vi "get_config.vi"(8 "error in":errorcluster) -> (0 "error out":errorcluster, 1 "key":string, 2 "model name":string, 3 "Provider Selector":enum32{"OpenAI", "Gemini"}(ring), 5 "proper config?":bool)   [LabVIEW 2020, in "lv_documentation.lvlib"]
uses:
  lv_documentation.lvlib
  <vilib>/Utility/config.llb/Read Key (String).vi
  <vilib>/Utility/config.llb/NI_LVConfig.lvlib
  <vilib>/httpClient/LabVIEWHTTPClient.lvlib
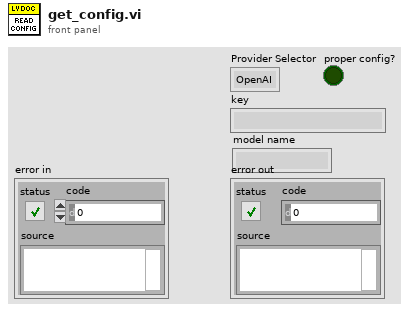
[diagram p1: front panel]
types:
  T1 = typedef "NI_LVConfig.lvlib/Config Data RefNum.ctl" = refnum<k1>
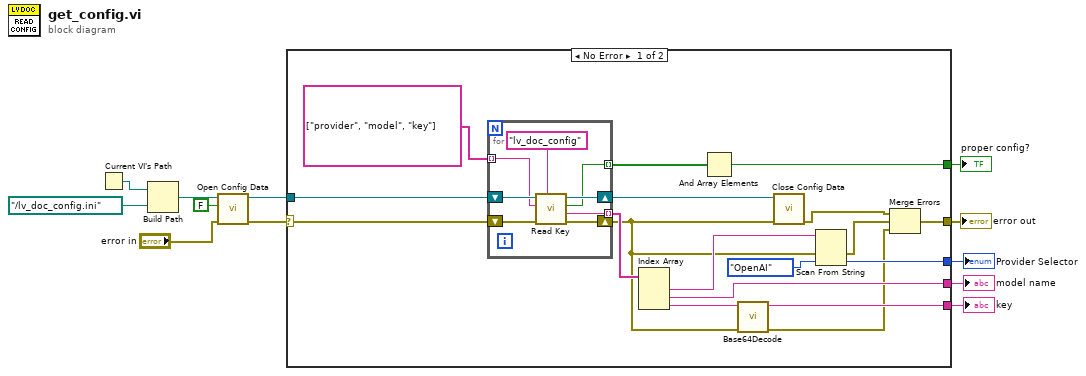
[diagram p0: block diagram]
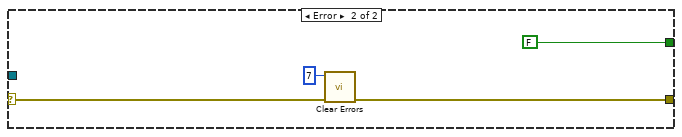
[diagram p2: hidden frame]
diagram:
  n1 = Current VI's Path() -> (path=w11:path)
  n2 = Build Path(base path=w11, name or relative path=path "../lv_doc_config.ini") -> (appended path=w8:path)
  n3 = call <vilib>:"Open Config Data.vi"("error in (no error)"="error in", "create file if necessary (T)"=FALSE, "configuration file path"=w8) -> ("error out"=w12:errorcluster, "refnum"=w9:T1)  [unwired: 6 in, 1 out]
  n4 = case shown="No Error" w12 {
    selector: w12 -> [w30 w42]
    tunnel: w9 -> [w29 _]
    tunnel: [w13 w40] -> w3
    tunnel: [w25 FALSE ("found?")] -> w2
    tunnel: [w22 _] -> w6
    tunnel: [w18 _] -> w5
    tunnel: [w17 _] -> w4
    frame No Error {
      n5 = for {
        shift-right: [w37] -> w19
        shift-left: w30 -> [w38]
        shift-right: [w35] -> w28
        shift-left: w29 -> [w36]
        tunnel: string[] ["provider", "model", "key"] ("appended array") -> [w33] mode=indexing
        tunnel: [w32] -> w26 mode=indexing
        tunnel: [w31] -> w24 mode=indexing
        n6 = call-poly <vilib>:"Read Key.vi"("section"="lv_doc_config", "error in (no error)"=w38, "key"=w33, "refnum"=w36) -> ("error out"=w37:errorcluster, "value"=w31:string, "found?"=w32:bool, "refnum out"=w35:T1)  [unwired: 4 in]
      }
      n7 = Index Array(array=w24) -> (element #1=w21:string, element #2=w17:string, element #3=w23:string)  [unwired: 3 in]
      n8 = And Array Elements(Boolean array=w26) -> (logical AND=w25:bool)
      n9 = call <vilib>:"Base64Decode.vi"("error in (no error)"=w19, "buffer in"=w23) -> ("error out"=w14:errorcluster, "decoded string"=w22:string)  [unwired: 8 in]
      n10 = call <vilib>:"Close Config Data.vi"("error in (no error)"=w19, "refnum"=w28) -> ("error out"=w16:errorcluster)  [unwired: 8 in, 1 out]
      n11 = Scan From String(input string=w21, error in=w19, default 1=enum32{"OpenAI", "Gemini"}."OpenAI" ("Provider Selector")) -> (error out=w15:errorcluster, output 1=w18:enum32{"OpenAI", "Gemini"})  [unwired: 2 in, 2 out]
      n12 = Merge Errors(w16, w15, w14) -> (w13:errorcluster)
    }
    frame Error {
      n13 = call <vilib>:"Clear Errors.vi"("error in (no error)"=w42, "specific error code to clear (0: all)"=7) -> ("error out"=w40:errorcluster)  [unwired: 4 in, 1 out]
    }
  }
  "Provider Selector" <- w5
  "key" <- w6
  "model name" <- w4
  "error out" <- w3
  "proper config?" <- w2
